vi "Set NVMEM Bytes.vi"(0 "session in":refnum<k21>, 1 "serial number":string, 2 "password":string, 5 "NVMEM area":refnum<k21>="$DefaultNVMEMAreas", 7 "data address":u32 format="%.0x", 9 "data":u8[](array[numeric]) format="%.0x", 11 "error in (no error)":errorcluster) -> (4 "session out":refnum<k21>, 6 "NVMEM area out":refnum<k21>, 8 "next data address":u32 format="%.0x", 15 "error out":errorcluster)   [LabVIEW 2020, in "SLSC.lvlib"]
doc: "Sets the bytes of <B>data</B> to be written to the <B>data address </B> in the specified <B>NVMEM area</B>. If you set the same address multiple times between commits, only the last value will be committed. Some areas in the NVMEM of an SLSC module may be protected. You need to specify a serial number and password to write to protected areas."
uses:
  <vilib>/SLSC/SLSC.lvlib
  nislsclvapi.dll
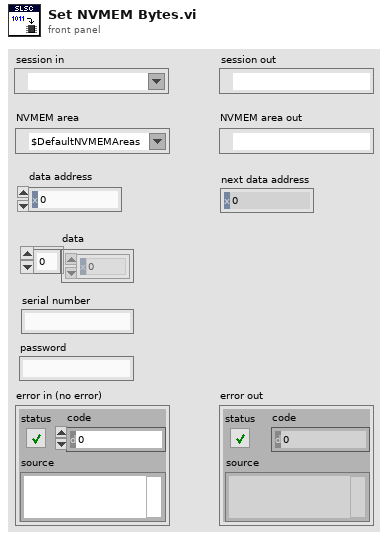
[diagram p1: front panel]
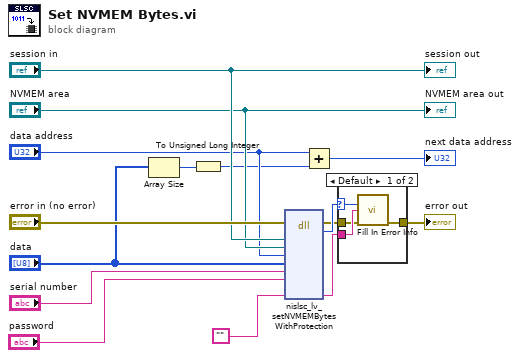
[diagram p0: block diagram]
diagram:
  n1 = Array Size(array="data") -> (size(s)=w4:i32)
  n2 = To Unsigned Long Integer(number=w4) -> (unsigned 32bit integer=w3:u32)
  n3 = dll-call lib="nislsclvapi.*" fn="nislsc_lv_setNVMEMBytesWithProtection"(error in="error in (no error)", "session"="session in", "nvmemArea"="NVMEM area", "registerAddress"="data address", "data"="data", "serialNum"="serial number", "password"="password", "extendedErrorInfo"="") -> (error out=w10:errorcluster, "return type"=w11:i32, "extendedErrorInfo"=w12:string)  [unwired: 10 in, 1 out]
  n4 = Add(x="data address", y=w3) -> (x+y=→"next data address":u32)
  n5 = case shown="Default" w11 {
    selector: w11 -> [w19 _]
    tunnel: w12 -> [w18 _]
    tunnel: w10 -> [w17 w20]
    tunnel: [w16 w20] -> w9
    frame Default {
      n6 = call <vilib>:"Fill In Error Info.vi"("status code"=w19, "extended error info"=w18, "error in"=w17) -> ("error out"=w16:errorcluster)  [unwired: 12 in]
    }
    frame 0 {
    }
  }
  "error out" <- w9
  "session out" <- "session in"
  "NVMEM area out" <- "NVMEM area"
